vi "GV-file-code.vi"(1 "offset":u32, 2 "string input":string) -> (0 "string output":string)   [LabVIEW 2020]
doc: "Code file (from ASCII)"
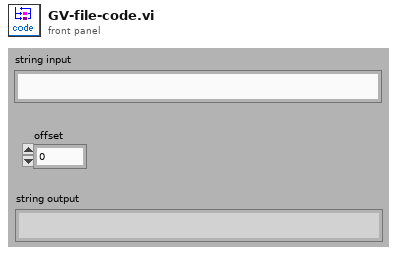
[diagram p1: front panel]
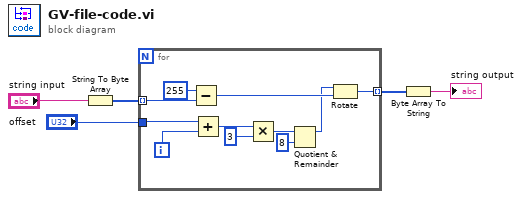
[diagram p0: block diagram]
diagram:
  n1 = String To Byte Array(string="string input") -> (unsigned byte array=w3:u8[])
  n2 = for {
    tunnel: "offset" -> [w16]
    tunnel: w3 -> [w14] mode=indexing
    tunnel: [w6] -> w2 mode=indexing
    i -> [w15]
    n3 = Subtract(x=u8 255, y=w14) -> (x-y=w8:u8)
    n4 = Add(x=w16, y=w15) -> (x+y=w12:u32)
    n5 = Multiply(x=w12, y=u32 3) -> (x*y=w10:u32)
    n6 = Quotient & Remainder(x=w10, y=u32 8) -> (x-y*floor(x/y)=w7:u32)  [unwired: 1 out]
    n7 = Rotate(1:w8, 2:w7) -> (0:w6:u8)
  }
  n8 = Byte Array To String(unsigned byte array=w2) -> (string=→"string output":string)
